vi "ZDataVIS_ScaleSelect.vi"(4 "Manual CTLs":T1={"X Low"=-0.1, "X High"=0.1, "X Step Size"=4e-05} {"X Step Size" format="%#_6p"; "X High" format="%#_6p"; "X Low" format="%#_6p"}, 6 "Auto CTLs":cluster{"METHOD":bool, "Steps":dbl}, 8 "error in (no error)":errorcluster, 10 "X Scale Selection 2":enum32{"Manual", "Auto"}(tab), 11 "Intensity Info IN":cluster{dbl[], dbl[]}[](array[cluster])) -> (0 "error out":errorcluster, 2 "X Step Info":cluster{"X Low":dbl, "X High":dbl, "X Step":dbl}={"X Low"=-0.1, "X High"=0.1, "X Step"=4e-05} {"X Step" format="%#_6p"; "X High" format="%#_6p"; "X Low" format="%#_6p"}, 3 "Intensity InfoOUT":cluster{dbl[], dbl[]}[](array[cluster]))   [LabVIEW 2016]
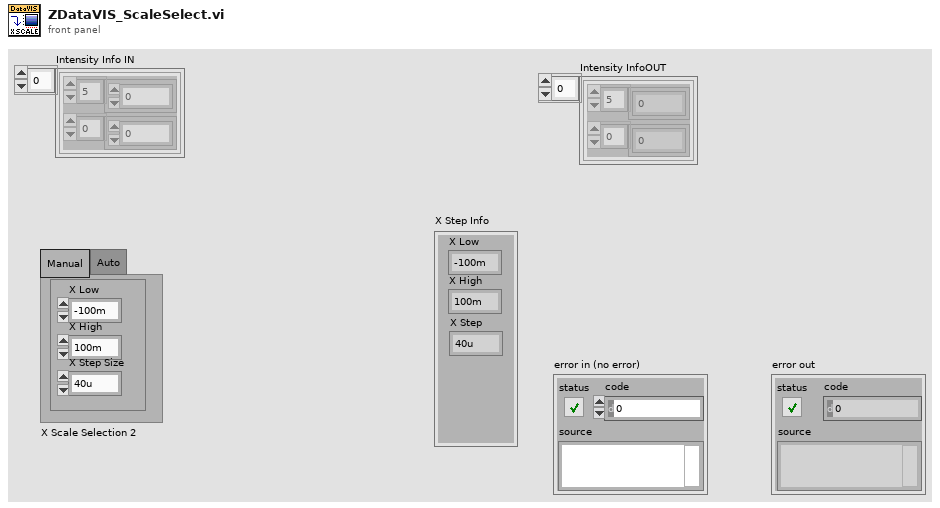
[diagram p1: front panel]
types:
  T1 = cluster{"X Low":dbl, "X High":dbl, "X Step Size":dbl}
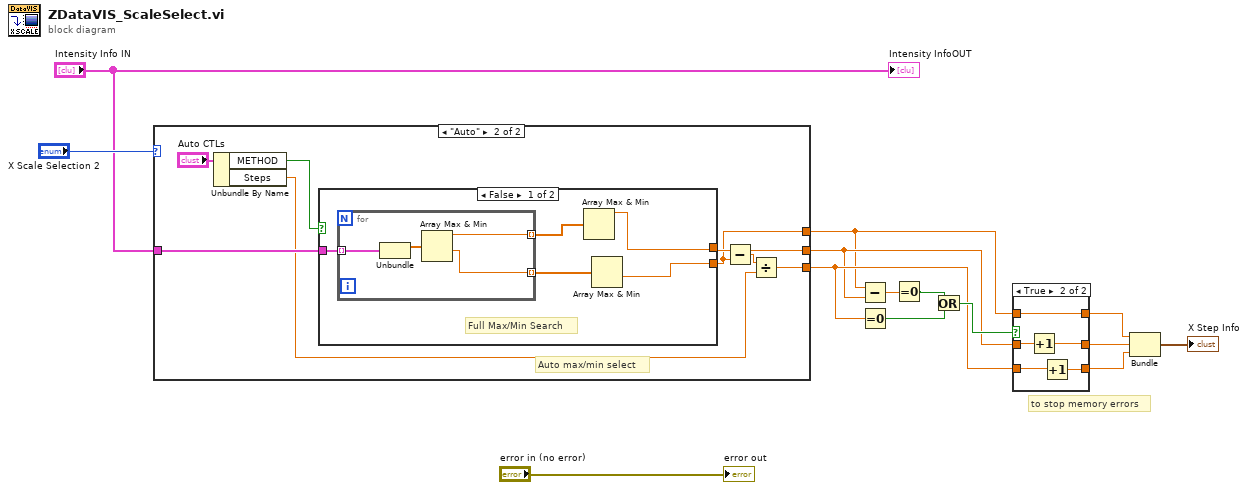
[diagram p0: block diagram]
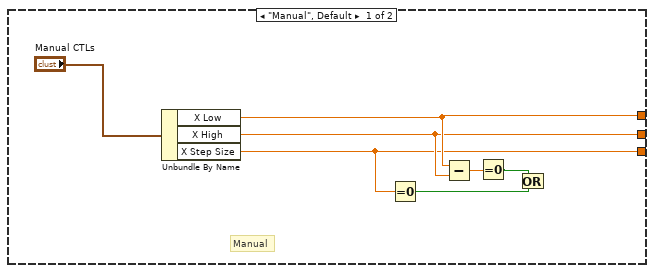
[diagram p3: hidden frame]
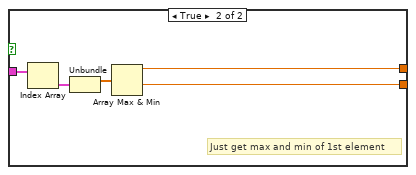
[diagram p4: hidden frame]
diagram:
  # "to stop memory errors"
  n1 = case shown="\"Auto\"" "X Scale Selection 2" {
    tunnel: [w17 w25] -> w6
    tunnel: [w20 w27] -> w4
    tunnel: [w19 w28] -> w5
    tunnel: "Intensity Info IN" -> [_ w29]
    frame "Manual", Default {
      # "Manual"
      n2 = Unbundle By Name("Manual CTLs") -> ("X Low"=w20:dbl, "X High"=w19:dbl, "X Step Size"=w17:dbl)
      n3 = Equal To 0?(x=w17) -> (x = 0?=w16:bool)
      n4 = Subtract(x=w20, y=w19) -> (x-y=w18:dbl)
      n5 = Equal To 0?(x=w18) -> (x = 0?=w15:bool)
      n6 = Or(x=w15, y=w16) -> ()  [unwired: 1 out]
    }
    frame "Auto" {
      # "Auto max/min select"
      n7 = Unbundle By Name("Auto CTLs") -> ("METHOD"=w23:bool, "Steps"=w22:dbl)
      n8 = case shown="False" w23 {
        tunnel: [w30 w40] -> w27
        tunnel: [w31 w39] -> w28
        tunnel: w29 -> [w34 w43]
        frame False {
          # "Full Max/Min Search"
          n9 = for {
            tunnel: w34 -> [w37] mode=indexing
            tunnel: [w36] -> w33 mode=indexing
            tunnel: [w35] -> w32 mode=indexing
            n10 = Unbundle(w37) -> (w38:dbl[])  [unwired: 1 out]
            n11 = Array Max & Min(array=w38) -> (max value=w36:dbl, min value=w35:dbl)  [unwired: 2 out]
          }
          n12 = Array Max & Min(array=w33) -> (max value=w31:dbl)  [unwired: 3 out]
          n13 = Array Max & Min(array=w32) -> (min value=w30:dbl)  [unwired: 3 out]
        }
        frame True {
          # "Just get max and min of 1st element"
          n14 = Index Array(array=w43) -> (element=w42:cluster{dbl[], dbl[]})  [unwired: 1 in]
          n15 = Unbundle(w42) -> (w41:dbl[])  [unwired: 1 out]
          n16 = Array Max & Min(array=w41) -> (max value=w39:dbl, min value=w40:dbl)  [unwired: 2 out]
        }
      }
      n17 = Subtract(x=w28, y=w27) -> (x-y=w26:dbl)
      n18 = Divide(x=w26, y=w22) -> (x/y=w25:dbl)
    }
  }
  n19 = Subtract(x=w4, y=w5) -> (x-y=w10:dbl)
  n20 = Equal To 0?(x=w6) -> (x = 0?=w9:bool)
  n21 = Equal To 0?(x=w10) -> (x = 0?=w8:bool)
  n22 = Or(x=w8, y=w9) -> (x .or. y?=w7:bool)
  n23 = case shown="True" w7 {
    tunnel: w6 -> [w44 w49]
    tunnel: w5 -> [w45 w51]
    tunnel: w4 -> [w46 w47]
    tunnel: [w46 w47] -> w3
    tunnel: [w45 w50] -> w2
    tunnel: [w44 w48] -> w1
    frame False {
    }
    frame True {
      n24 = Increment(x=w51) -> (x+1=w50:dbl)
      n25 = Increment(x=w49) -> (x+1=w48:dbl)
    }
  }
  n26 = Bundle("X Low"=w3, "X High"=w2, "X Step Size"=w1) -> (→"X Step Info":T1)  [unwired: 1 in]
  "error out" <- "error in (no error)"
  "Intensity InfoOUT" <- "Intensity Info IN"
